vi "DC Voltmeter (Express).vi"() -> ()   [LabVIEW 2015]
panel:
  out "error out":errorcluster
  in  "stop":bool
  out "Voltage":dbl
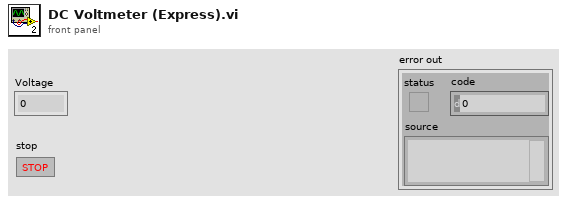
[diagram p1: front panel]
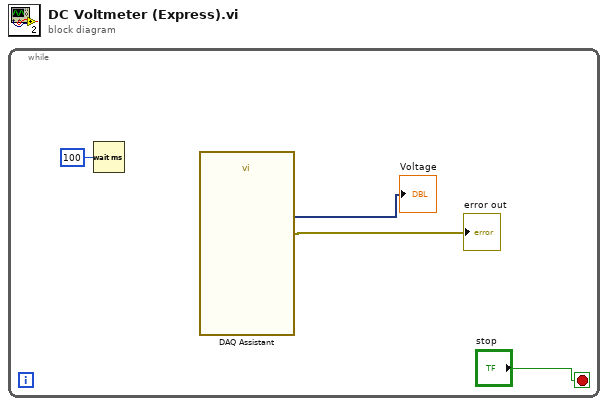
[diagram p0: block diagram]
diagram:
  n1 = while {
    stop <- "stop" stop-if-true
    n2 = Wait (ms)(milliseconds to wait=u32 100) -> ()  [unwired: 1 out]
    n3 = call "DAQ Assistant"() -> ("data"=→"Voltage":dynamicdata, "error out"=→"error out":errorcluster)  [unwired: 17 in, 1 out]
  }
